vi "Create_Scan_comment_string.vi"(1 "Requested channels":i32[](array[numeric]), 2 "Scan comments":string[](array[string])) -> (0 "Comment string":string)   [LabVIEW 2014]
uses:
  ADAM_Global.vi
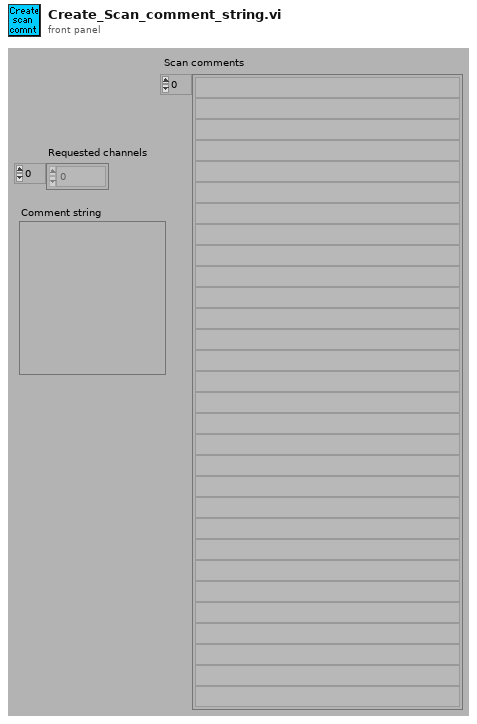
[diagram p1: front panel]
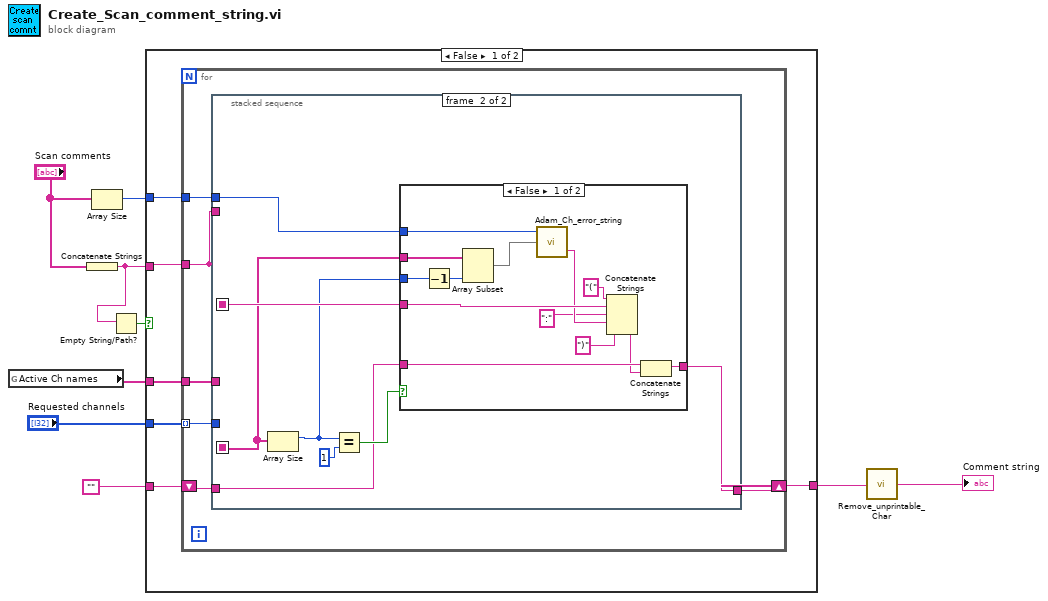
[diagram p0: block diagram]
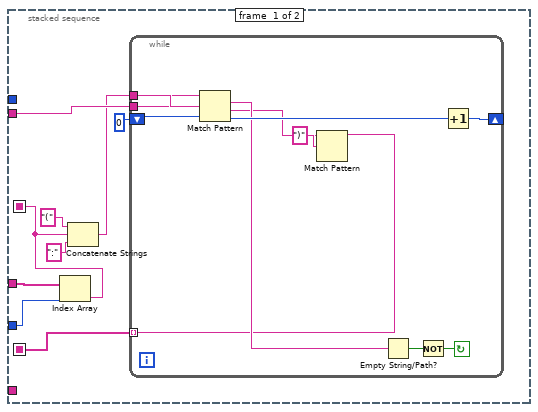
[diagram p2: hidden frame]
diagram:
  n1 = global read "ADAM_Global.vi" "Active Ch names"() -> (w8:string[])
  n2 = Concatenate Strings("Scan comments") -> (w6:string)
  n3 = Array Size(array="Scan comments") -> (size(s)=w3:i32)
  n4 = Empty String/Path?(string/path=w6) -> (empty?=w5:bool)
  n5 = case shown="False" w5 {
    tunnel: "Requested channels" -> [w15 _]
    tunnel: w8 -> [w14 _]
    tunnel: [w13 w64] -> w2
    tunnel: "" -> [w12 w64]
    tunnel: w6 -> [w11 _]
    tunnel: w3 -> [w10 _]
    frame False {
      n6 = for {
        tunnel: w15 -> [w21] mode=indexing
        tunnel: w14 -> [w20]
        tunnel: [w19] -> _ mode=indexing
        shift-right: [w17] -> w13
        shift-left: w12 -> [w18]
        tunnel: w11 -> [w19]
        tunnel: w10 -> [w16]
        n7 = stacked-sequence {
          seq-local: [w25 _] -> [_ w45]
          seq-local: [w23 _] -> [_ w43]
          tunnel: w21 -> [w22 _]
          tunnel: w20 -> [w30 _]
          tunnel: w19 -> [w29 _]
          tunnel: w18 -> [_ w47]
          tunnel: [_ w46] -> w17
          tunnel: w16 -> [_ w44]
          frame #0 {
            n8 = Index Array(array=w30, index=w22) -> (element=w25:string)
            n9 = Concatenate Strings("(", w25, ":") -> (w24:string)
            n10 = while {
              tunnel: [w31] -> w23 mode=indexing
              shift-left: 0 ("offset past match") -> [w35]
              shift-right: [w36] -> _
              tunnel: w29 -> [w40]
              tunnel: w24 -> [w41]
              stop <- w37 continue-if-true
              n11 = Match Pattern(string=w40, regular expression=w41, offset (0)=w35) -> (match substring=w33:string, after substring=w32:string, offset past match=w39:i32)  [unwired: 1 out]
              n12 = Match Pattern(string=w32, regular expression=")" ("String to match")) -> (before substring=w31:string)  [unwired: 4 out]
              n13 = Empty String/Path?(string/path=w33) -> (empty?=w38:bool)
              n14 = Not(x=w38) -> (.not. x?=w37:bool)
              n15 = Increment(x=w39) -> (x+1=w36:i32)
            }
          }
          frame #1 {
            n16 = Array Size(array=w43) -> (size(s)=w42:i32)
            n17 = Equal?(x=w42, y=1) -> (x = y?=w48:bool)
            n18 = case shown="False" w48 {
              tunnel: w45 -> [w61 _]
              tunnel: w47 -> [w60 w63]
              tunnel: [w58 w63] -> w46
              tunnel: w44 -> [w54 _]
              tunnel: w43 -> [w51 _]
              tunnel: w42 -> [w50 _]
              frame False {
                n19 = Decrement(x=w50) -> (x-1=w53:i32)
                n20 = Array Subset(array=w51, length=w53) -> (w52:string[])  [unwired: 1 in]
                n21 = call "Adam_Ch_error_string.vi"("String array"=w52, "Number of scans"=w54) -> ("Comment string"=w57:string)  [unwired: 2 out]
                n22 = Concatenate Strings("(", w61, ":", w57, ")") -> (w59:string)
                n23 = Concatenate Strings(w60, w59) -> (w58:string)
              }
              frame True {
              }
            }
          }
        }
      }
    }
    frame True {
    }
  }
  n24 = call "Remove_unprintable_Char.vi"("Input String"=w2) -> ("Output String"=→"Comment string":string)
